vi "Get CalDate.vi"() -> (3 "LastCalDate":string=" 5- 6-2012")   [LabVIEW 2015]
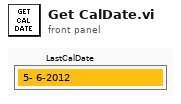
[diagram p1: front panel]
types:
  T1 = typedef "LVDateTimeRec.ctl" = cluster{"fractional second":dbl, "second":i32, "minute":i32, "hour":i32, "day of month":i32, "month":i32, "year":i32, "day of week":i32, "day of year":i32, "DST":i32}
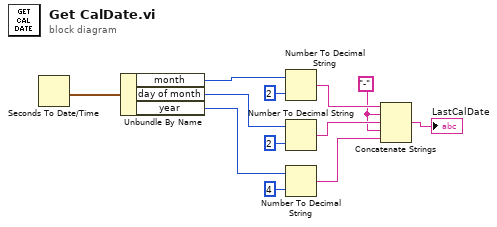
[diagram p0: block diagram]
diagram:
  w2 = "-"
  n1 = Seconds To Date/Time() -> (date time rec=w12:T1)  [unwired: 2 in]
  n2 = Unbundle By Name(w12) -> ("month"=w11:i32, "day of month"=w8:i32, "year"=w6:i32)
  n3 = Number To Decimal String(number=w11, width (-)=i16 2) -> (decimal integer string=w5:string)
  n4 = Number To Decimal String(number=w8, width (-)=i16 2) -> (decimal integer string=w4:string)
  n5 = Number To Decimal String(number=w6, width (-)=i16 4) -> (decimal integer string=w3:string)
  n6 = Concatenate Strings(w5, w2, w4, w2, w3) -> (→"LastCalDate":string)
